vi "FRCts20_WebMethods_Request_GET.vi"(7 "httpRequestID":u32, 10 "RequestUniqueId":string="-1") -> ()   [LabVIEW 2014, in "FRCts20_WebMethods.lvlib"]
doc: "<B>GET</B> on the specified <B>request</B> resource\n\nIf request is not specified, will return all resources. Requests can be filtered using the following parameters in the query string:\n - <B>division</B>\n - <B>team</B>\n - <B>status</B> (Open, In Work, Closed)\n\nhttp://<server address>:<port>/FRCts/request/<B>request</B>"
uses:
  FRCts20_WebMethods.lvlib
  Backend/source/VI Source/FRCts20_Backend_API/FRCts20_Backend_API.lvlib
  Backend/source/VI Source/FRCts20_Backend_API/FRCts20_Backend_API_Status.ctl
  Backend/source/VI Source/FRCts20_Backend_API/FRCts20_Backend_API_Request.vi
  Backend/source/VI Source/FRCts20_Backend_API/FRCts20_Backend_API_Request.ctl
  ESP Engine/source/VI Source/FRCts20_EspEngine.lvlib
  Backend/source/VI Source/FRCts20_Backend_API/FRCts20_Backend_API_Command_Request.ctl
  Backend/source/VI Source/FRCts20_Backend_API/FRCts20_Backend_API_Team.vi
  Backend/source/VI Source/FRCts20_Backend_API/FRCts20_Backend_API_SW.ctl
  Backend/source/VI Source/FRCts20_Backend_API/FRCts20_Backend_API_Team.ctl
  Backend/source/VI Source/FRCts20_Backend_API/FRCts20_Backend_API_Command_Team.ctl
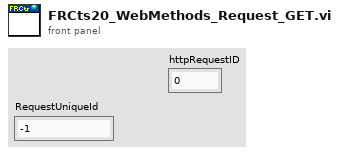
[diagram p1: front panel]
types:
  T1 = typedef "FRCts20_Backend_API.lvlib/FRCts20_Backend_API_Command_Team.ctl" = string
  T2 = typedef "FRCts20_Backend_API.lvlib/FRCts20_Backend_API_Team.ctl" = cluster{"Team Index":u32, "Team Number":u32, "Team Name":string, "Short Team Name":string, "Nick Name":string, "Robot Name":string, "City":string, "State":string, "Country":string, "Rookie Year":u32, "SWType":T3, "CAN":bool, "Vision":bool, "Kinect":bool, "Tags":string, "Avatar":string, "Request Array":cluster{"Request Index":u32, "Description":string, "Status":T4, "Open Date":timestamp, "Last Update":timestamp, "Close Date":timestamp}[], "Events Attending":cluster{"EventIndex":dbl, "EventName":string, "IsLive":bool}[], "APIReturn":string}
  T3 = typedef "FRCts20_Backend_API.lvlib/FRCts20_Backend_API_SW.ctl" = string
  T4 = typedef "FRCts20_Backend_API.lvlib/FRCts20_Backend_API_Status.ctl" = enum16{"Open", "In Work", "Closed"}
  T5 = typedef "FRCts20_Backend_API.lvlib/FRCts20_Backend_API_Command_Request.ctl" = string
  T6 = typedef "FRCts20_Backend_API.lvlib/FRCts20_Backend_API_Request.ctl" = cluster{"Request Index":u32, "Description":string, "Status":T4, "Open Date":timestamp, "Last Update":timestamp, "Closed Date":timestamp, "Notes":cluster{"Note Index":u32, "Text":string, "Time Entered":timestamp, "Author":string, "Solution":bool}[], "Team Index":u32, "APIReturn":string}
  T7 = typedef "FRCts20_EspEngine.lvlib/FRCts20_EspEngine_SearchBrowser.ctl" = cluster{"Event":cluster{"Event Index":u32, "Event Name":string, "Start Time":timestamp, "End Time":timestamp, "OpenIssues":u8, "IsLive":bool}[], "select-choice-software":string, "select-choice-location":string}
  T8 = typedef "FRCts20_EspEngine.lvlib/FRCts20_EspEngine_Request.ctl" = cluster{"Request":T9, "CommentListLength":i16}
  T9 = typedef "FRCts20_WebMethods.lvlib/FRCts20_WebMethods_ctl_request.ctl" = cluster{"Event":string, "Description":string, "Status":T4, "Open Date":string, "Last Update":string, "Close Date":string, "UniqueId":i32, "Team":cluster{"Team Nickname":string, "Team Number ":i32, "UniqueId":i32}, "Comments":cluster{"Request Number":dbl, "Text":string, "Author":string, "IsSolution":bool, "Team":cluster{"Team Nickname":string, "Team Identifier ":dbl}, "UniqueId":i32}[]}
  T10 = typedef "FRCts20_EspEngine.lvlib/FRCts20_EspEngine_Team.ctl" = cluster{"Team":T11, "RequestListLength":i16, "Requests":T9[]}
  T11 = typedef "FRCts20_WebMethods.lvlib/FRCts20_WebMethods_ctl_singleTeam.ctl" = cluster{"Events":string[], "Robot Name":string, "Kinect":bool, "Vision":bool, "Can":bool, "Tags":string, "Avatar URL":string, "Team":T12, "SWType":T3}
  T12 = typedef "FRCts20_WebMethods.lvlib/FRCts20_WebMethods_ctl_teamIdentifier.ctl" = cluster{"Team Nickname":string, "Team Number ":u32, "UniqueId":u32}
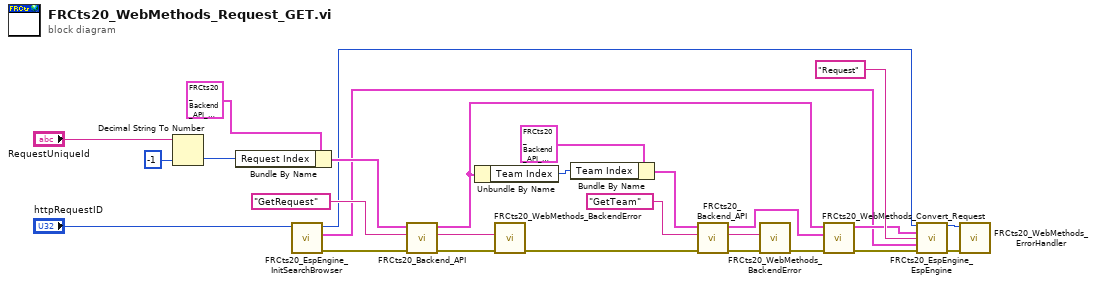
[diagram p0: block diagram]
diagram:
  n1 = Decimal String To Number(string="RequestUniqueId", default (0L)=i64 -1 ("default (0 I32)")) -> (number=w22:i64)  [unwired: 1 in, 1 out]
  n2 = Bundle By Name(cluster=T6 {"Request Index"=0, "Description"="", "Status"=enum."Open", "Open Date"=timestamp(0 s since 1904-01-01), "Last Update"=timestamp(0 s since 1904-01-01), "Closed Date"=timestamp(0 s since 1904-01-01), "Notes"=[], "Team Index"=0, "APIReturn"=""} ("Request In"), "Request Index"=w22) -> (w21:T6)
  n3 = call "FRCts20_EspEngine_InitSearchBrowser.vi"("httpRequestID"="httpRequestID") -> ("error out"=w4:errorcluster, "SearchBrowser"=w1:T7, "httpRequestID out"=w2:u32)  [unwired: 8 in]
  n4 = call-poly "FRCts20_Backend_API.vi"("error in (no error)"=w4, "Command"=T5 "GetRequest", "Request In"=w21) -> ("error out"=w25:errorcluster, "Status"=w26:string, "Request Out"=w7:T6)  [unwired: 6 in]
  n5 = Unbundle By Name(w7) -> ("Team Index"=w6:u32)
  n6 = call "FRCts20_WebMethods_BackendError.vi"("error in (no error)"=w25, "Status"=w26) -> ("error out"=w14:errorcluster)  [unwired: 8 in, 1 out]
  n7 = Bundle By Name(cluster=T2 {"Team Index"=0, "Team Number"=0, "Team Name"="", "Short Team Name"="", "Nick Name"="", "Robot Name"="", "City"="", "State"="", "Country"="", "Rookie Year"=0, "SWType"="", "CAN"=FALSE, "Vision"=FALSE, "Kinect"=FALSE, "Tags"="", "Avatar"="", "Request Array"=[], "Events Attending"=[], "APIReturn"=""} ("Team In"), "Team Index"=w6) -> (w12:T2)
  n8 = call-poly "FRCts20_Backend_API.vi"("error in (no error)"=w14, "Command"=T1 "GetTeam", "Team In"=w12) -> ("error out"=w10:errorcluster, "Status"=w9:string, "Team Out"=w5:T2)  [unwired: 6 in]
  n9 = call "FRCts20_WebMethods_BackendError.vi"("error in (no error)"=w10, "Status"=w9) -> ("error out"=w8:errorcluster)  [unwired: 8 in, 1 out]
  n10 = call "FRCts20_WebMethods_Convert_Request.vi"("error in (no error)"=w8, "Team Out"=w5, "Request Out"=w7) -> ("error out"=w15:errorcluster, "Request+Team"=w16:cluster{"Request":T8, "Team":T10})  [unwired: 7 in]
  n11 = call "FRCts20_EspEngine_EspEngine.vi"("httpRequestID"=w2, "Cluster"=w16, "Page"="Request", "SearchBrowser"=w1, "error in (no error)"=w15) -> ("httpRequestID out"=w19:u32, "error out"=w20:errorcluster)  [unwired: 9 in]
  n12 = call "FRCts20_WebMethods_ErrorHandler.vi"("error in"=w20, "httpRequestID"=w19) -> ()  [unwired: 9 in, 1 out]
